vi "Get PString.vi"(2 "offset(0)":i32, 3 "String":string) -> (0 "offset  Past PString":i32, 1 "PString":string)   [LabVIEW 2012, in "TD Tools.lvlib"]
uses:
  TD Tools.lvlib
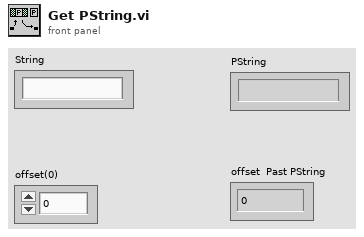
[diagram p1: front panel]
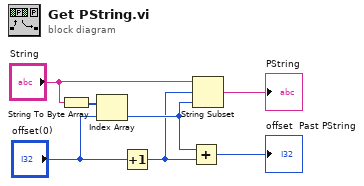
[diagram p0: block diagram]
diagram:
  n1 = String To Byte Array(string="String") -> (unsigned byte array=w5:u8[])
  n2 = Index Array(array=w5, index="offset(0)") -> (element=w7:u8)
  n3 = Increment(x="offset(0)") -> (x+1=w6:i32)
  n4 = Add(x=w7, y=w6) -> (x+y=→"offset  Past PString":i32)
  n5 = String Subset(string="String", offset (0)=w6, length (rest)=w7) -> (substring=→"PString":string)
